vi "Request Data JSON.vi"(8 "error in (no error)":errorcluster, 11 "GetInputList in":refnum<class "GetInputList.lvclass">) -> (0 "error out":errorcluster, 2 "Request Data JSON":string, 3 "GetInputList out":refnum<class "GetInputList.lvclass">)   [LabVIEW 2022 SP3, in "obs-websocket-lv.lvlib" / "GetInputList.lvclass"]
uses:
  GetInputList.lvclass
  GetInputList.lvclass/GetInputList.ctl
  <vilib>/IlluminatedG/lv-web-crypto/lv-json/JSON/JSON.lvlib
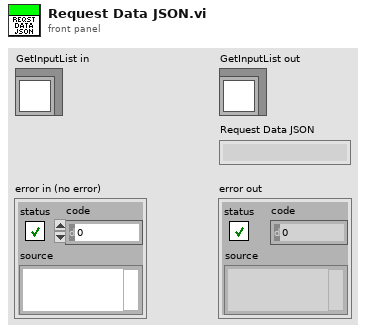
[diagram p1: front panel]
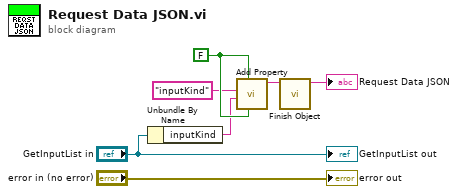
[diagram p0: block diagram]
diagram:
  w4 = FALSE ("Include Empty?")
  n1 = Unbundle By Name("GetInputList in") -> ("inputKind"=w1:string)
  n2 = call <vilib>:"Add Property.vi"("String?"=w4, "Include Empty?"=w4, "Value"=w1, "Property Name"="inputKind") -> ("String out"=w6:string)  [unwired: 7 in]
  n3 = call <vilib>:"Finish Object.vi"("String In"=w6) -> ("String out"=→"Request Data JSON":string)  [unwired: 10 in]
  "error out" <- "error in (no error)"
  "GetInputList out" <- "GetInputList in"
